vi "Is Valid.vi"(11 "Error Interface in":refnum<class "Error Interface.lvclass">) -> (3 "Error Interface out":refnum<class "Error Interface.lvclass">, 4 "Valid?":bool)   [LabVIEW 2016, in "Stream Error.lvlib" / "Error Interface.lvclass"]
doc: "--\nCopyright © 2017 Composed SystemsI All rights reserved.\n\nAuthor: Jon McBee <jon.mcbee@composed.io>\n\nThis library is provided \"AS IS\" ,WITHOUT WARRANTIES OR\nCONDITIONS OF ANY KIND, either express or implied.\n\nComposed Systems -- composed.io\n\nStream 0.0.1.1\nJon McBee - Composed Systems\nCopyright (c) 2017, Composed Systems"
uses:
  <userlib>/Composed Systems/Stream/Error/Classes/Error Interface/Error Interface.lvclass
  <userlib>/Composed Systems/Stream/Error/Classes/Error Interface/Error Interface.lvclass/Error Interface.ctl
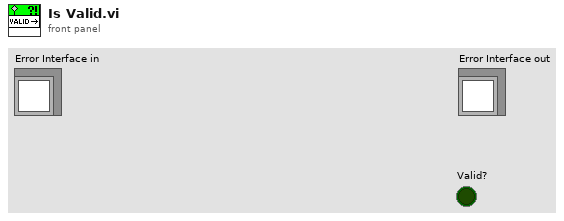
[diagram p1: front panel]
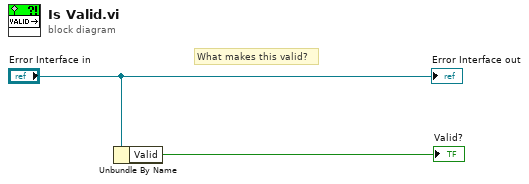
[diagram p0: block diagram]
diagram:
  # "What makes this valid?"
  n1 = Unbundle By Name("Error Interface in") -> ("Valid"=→"Valid?":bool)
  "Error Interface out" <- "Error Interface in"
